vi "Read.vi"(8 "error in (no error)":errorcluster, 11 "Numeric in":refnum<class "Const_I8_1D.lvclass">) -> (0 "error out":errorcluster, 2 "Numeric":T1, 3 "Numeric out":refnum<class "Const_I8_1D.lvclass">)   [LabVIEW 2021, in "Const_I8_1D.lvclass"]
uses:
  Const_I8_1D.lvclass
  Type.ctl
  Const_I8_1D.lvclass/Const_I8_1D.ctl
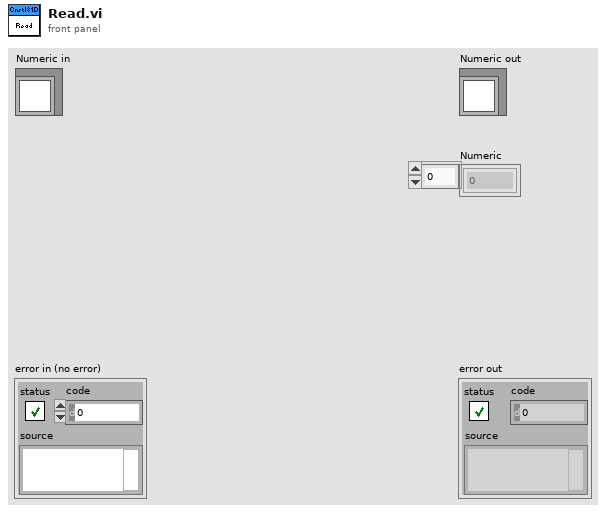
[diagram p1: front panel]
types:
  T1 = typedef "Const_I8_1D.lvclass/Type.ctl" = i8[]
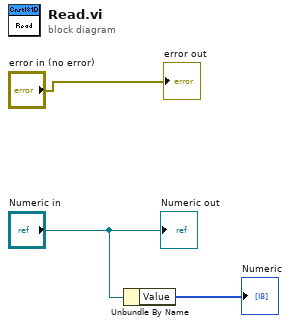
[diagram p0: block diagram]
diagram:
  n1 = Unbundle By Name("Numeric in") -> ("Value"=→"Numeric":T1)
  "error out" <- "error in (no error)"
  "Numeric out" <- "Numeric in"
